vi "Find Firmware Path.vi"(8 "error in":errorcluster, 10 "Device Class":string, 11 "Product ID":i32) -> (0 "error out":errorcluster, 3 "Firmware Path":path)   [LabVIEW 2020]
doc: "Retrieves the firmware path for the RT device."
uses:
  <vilib>/Utility/sysdir.llb/System Directory Type.ctl
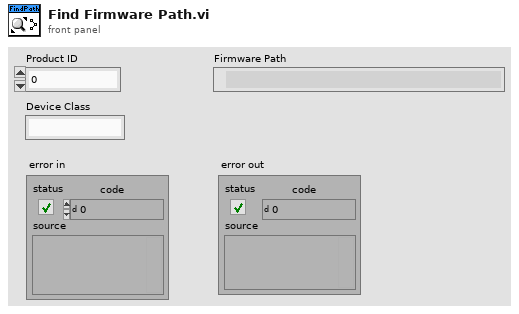
[diagram p1: front panel]
types:
  T1 = typedef "System Directory Type.ctl" = i32
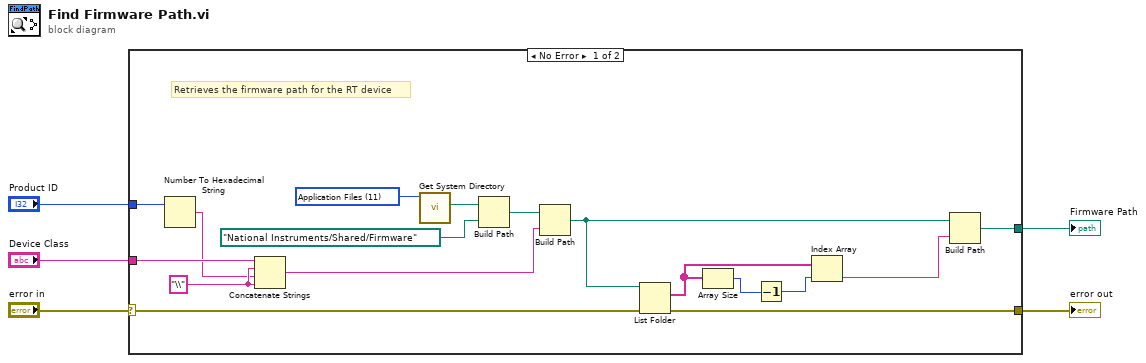
[diagram p0: block diagram]
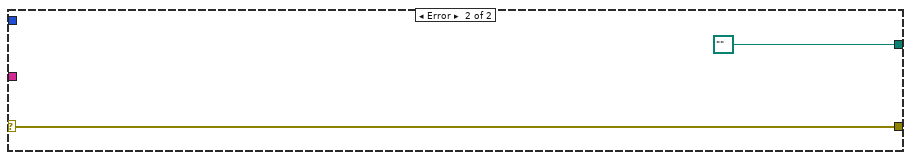
[diagram p2: hidden frame]
diagram:
  n1 = case shown="No Error" "error in" {
    selector: "error in" -> [w13 w24]
    tunnel: [w6 path "" ("appended path")] -> w5
    tunnel: [w11 w24] -> w3
    tunnel: "Product ID" -> [w19 _]
    tunnel: "Device Class" -> [w17 _]
    frame No Error {
      w18 = "\\"
      w20 = T1 11 items=["User Home"=0, "User Desktop"=1, "User Documents"=2, "User Application Data"=3, "User Preferences"=4, "User Temporary"=5, "Public Documents"=6, "Public Application Data"=7, "Public Preferences"=8, "Public Cache"=13, "System Core Libraries"=9, "System Installed Libraries"=10, "Application Files"=11, "Boot Volume Root"=12] ("system directory type")
      # "Retrieves the firmware path for the RT device"
      n2 = Number To Hexadecimal String(2:w19) -> (0:w16:string)  [unwired: 1 in]
      n3 = Concatenate Strings(w17, w18, w16, w18) -> (w14:string)
      n4 = call <vilib>:"Get System Directory.vi"("system directory type"=w20) -> ("system directory"=w21:path)  [unwired: 10 in]
      n5 = Build Path(base path=w21, name or relative path=path "National Instruments/Shared/Firmware") -> (appended path=w15:path)
      n6 = Build Path(base path=w15, name or relative path=w14) -> (appended path=w8:path)
      n7 = List Folder(path=w8, error in=w13) -> (filenames=w12:string[], error out=w11:errorcluster)  [unwired: 2 in, 2 out]
      n8 = Array Size(array=w12) -> (size(s)=w10:i32)
      n9 = Decrement(x=w10) -> (x-1=w9:i32)
      n10 = Index Array(array=w12, index=w9) -> (element=w7:string)
      n11 = Build Path(base path=w8, name or relative path=w7) -> (appended path=w6:path)
    }
    frame Error {
    }
  }
  "Firmware Path" <- w5
  "error out" <- w3
